vi "resize FP.vi"(4 "Width":u32, 6 "Screen Coordinates":T1, 7 "vi ref":refnum<vi>, 8 "error in (no error)":errorcluster, 11 "Loop data in":T2={"Config"={"List"=[], "max rows"=8, "Listbox placement"=enum."None", "String Color Options"={"Use? (F)"=FALSE, "Color - Valid"=0, "Color - Invalid"=0, "Allow blank?"=FALSE}}, "Refs"={"String"=refnum, "Listbox"=refnum}, "State"={"LB active?"=FALSE}}) -> (0 "error out":errorcluster, 3 "Loop data out":T2={"Config"={"List"=[], "max rows"=8, "Listbox placement"=enum."None", "String Color Options"={"Use? (F)"=FALSE, "Color - Valid"=0, "Color - Invalid"=0, "Allow blank?"=FALSE}}, "Refs"={"String"=refnum, "Listbox"=refnum}, "State"={"LB active?"=FALSE}})   [LabVIEW 2021, in "Autocomplete popup.lvlib"]
uses:
  Autocomplete popup.lvlib
  Autocomplete Textbox/SubVIs/Loop Data.ctl
  Autocomplete Textbox/SubVIs/Inputs.ctl
  Autocomplete Textbox/Classes/Handle/Listbox placement.ctl
  Autocomplete Textbox/SubVIs/Color String Options.ctl
  Autocomplete Textbox/SubVIs/Refs.ctl
  Autocomplete Textbox/SubVIs/State data.ctl
  <vilib>/Utility/miscctls.llb/LVPointTypeDef.ctl
  Autocomplete Textbox/Classes/Handle/Handle.lvclass
  Autocomplete Textbox/Autocomplete Textbox.lvlib
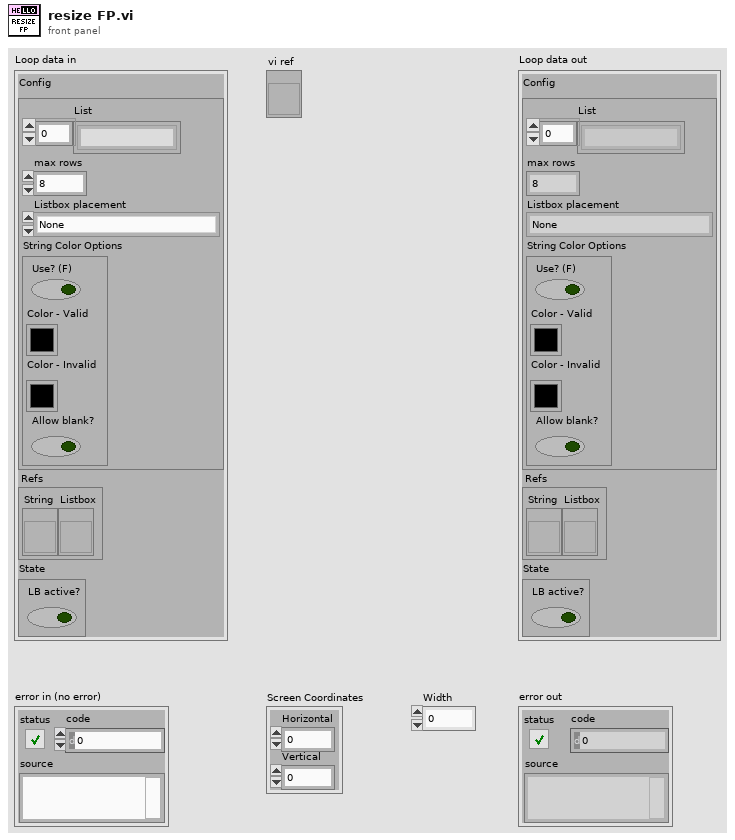
[diagram p1: front panel]
types:
  T1 = typedef "LVPointTypeDef.ctl" = cluster{"Horizontal":i16, "Vertical":i16}
  T2 = typedef "Autocomplete Textbox.lvlib/Loop Data.ctl" = cluster{"Config":T3, "Refs":T6, "State":T7}
  T3 = typedef "Autocomplete Textbox.lvlib/Inputs.ctl" = cluster{"List":string[], "max rows":i32, "Listbox placement":T4, "String Color Options":T5}
  T4 = typedef "Autocomplete Textbox.lvlib/Handle.lvclass/Listbox placement.ctl" = enum16{"None", "Under String", "Fit to Pane"}
  T5 = typedef "Autocomplete Textbox.lvlib/Color String Options.ctl" = cluster{"Use? (F)":bool, "Color - Valid":u32, "Color - Invalid":u32, "Allow blank?":bool}
  T6 = typedef "Autocomplete Textbox.lvlib/Refs.ctl" = cluster{"String":refnum<vi>, "Listbox":refnum<vi>}
  T7 = typedef "Autocomplete Textbox.lvlib/State data.ctl" = cluster{"LB active?":bool}
  T8 = typedef "LVRectTypeDef.ctl" = cluster{"Left":i16, "Top":i16, "Right":i16, "Bottom":i16}
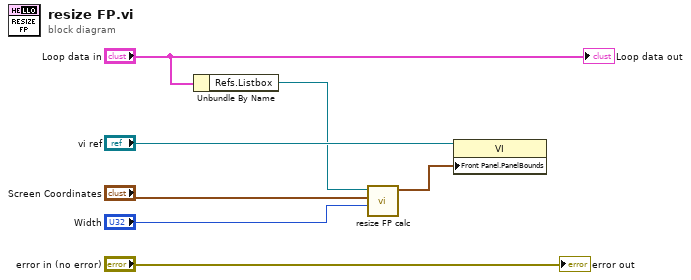
[diagram p0: block diagram]
diagram:
  n1 = Unbundle By Name("Loop data in") -> ("Refs.Listbox"=w4:refnum<vi>)
  n2 = call "resize FP calc.vi"("Width"="Width", "Screen Coordinates"="Screen Coordinates", "refs.listbox"=w4) -> ("fp bounds"=w1:T8)  [unwired: 8 in]
  n3 = property class="VI"(reference="vi ref", "Front Panel.PanelBounds"=w1) -> ()  [unwired: 1 in, 2 out]
  "Loop data out" <- "Loop data in"
  "error out" <- "error in (no error)"
